vi "Example NamedBundler 1.vi"() -> ()   [LabVIEW 2018]
uses:
  UserDefined StructType.ctl
panel:
  out "Error Out":errorcluster
  in  "Error In":errorcluster
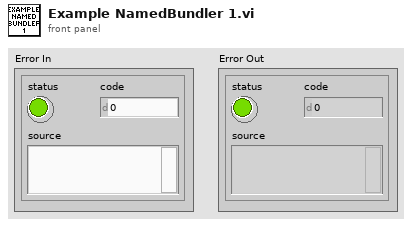
[diagram p1: front panel]
types:
  T1 = typedef "UserDefined StructType.ctl" = cluster{"LuboString":string, "NumInsideUserCluter":i32, "Double insideCluster":dbl}
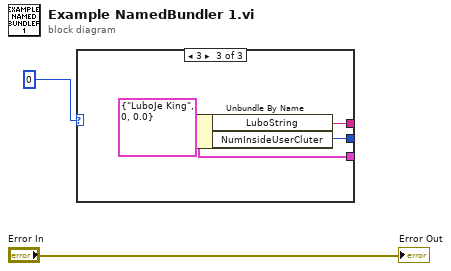
[diagram p0: block diagram]
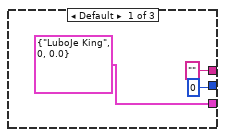
[diagram p2: hidden frame]
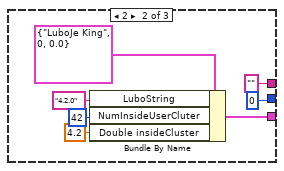
[diagram p3: hidden frame]
diagram:
  n1 = case shown="3" 0 {
    tunnel: [T1 {"LuboString"="LuboJe King", "NumInsideUserCluter"=0, "Double insideCluster"=0.0} ("totoSomNapisalLenTakSVK") w8 w15] -> _
    tunnel: ["" ("LuboString") "" ("LuboString") w14] -> _
    tunnel: [0 ("NumInsideUserCluter") 0 ("NumInsideUserCluter") w13] -> _
    frame Default {
    }
    frame 2 {
      n2 = Bundle By Name(cluster=T1 {"LuboString"="LuboJe King", "NumInsideUserCluter"=0, "Double insideCluster"=0.0} ("totoSomNapisalLenTakSVK"), "LuboString"="4.2.0", "NumInsideUserCluter"=42, "Double insideCluster"=4.2) -> (w8:T1)
    }
    frame 3 {
      w15 = T1 {"LuboString"="LuboJe King", "NumInsideUserCluter"=0, "Double insideCluster"=0.0} ("totoSomNapisalLenTakSVK")
      n3 = Unbundle By Name(w15) -> ("LuboString"=w14:string, "NumInsideUserCluter"=w13:i32)
    }
  }
  "Error Out" <- "Error In"
